vi "Charging_IPG Charging Status.vi"(8 "error in":errorcluster, 11 "MICS Dongle Address":refnum<visa-resource-name>="COM5") -> (0 "error out":errorcluster, 1 "IPG_ReceivedLevel":dbl=nan, 2 "TemperatureLevel":dbl=nan, 3 "ChargingState":string)   [LabVIEW 2010]
uses:
  Telemetry/Typedef Command List.ctl
panel:
  out "Charging Status":string
  out "ChargeWarning":dbl=nan
  # "Get Telemetry from IPG"
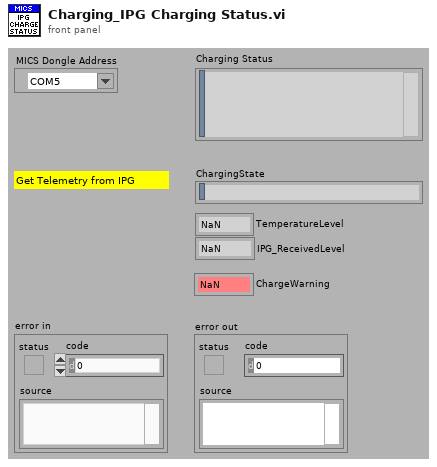
[diagram p1: front panel]
types:
  T1 = typedef "Typedef Command List.ctl" = enum16{"Get xPG Status", "xPG Stimulation", "Select Program", "Increment Program Amplitude", "Decrement Program Amplitude", "Get PoP Constants", "Get PPC Constants", "Get Program Names", "Set Pulse Amplitude", "Increment Pulse Amplitude", "Decrement Pulse Amplitude", "Get Pulse Widths", "Set Pulse Widths", "Increment Pulse Width", "Decrement Pulse Width", "Get Program Frequency", "Set Program Frequency", "Increment Program Frequency", "Decrement Program Frequency", "Inject Event", "Charging Control", "Get xPG Identity", "Set xPG Identity", "Restore Program Defaults", "Get Program Definition", "Set Program Definition", "Get Program Constants", "Set Program Constants", "Get Configurable Device Parameters", "Set Configurable Device Parameters", "Get Pulse Constants", "Set Pulse Constants", "Get Lead Limits", "Set Lead Limits", "Get Channel Calibrations", "Set Channel Calibrations", "<reserved 2>", "<reserved 3>", "<reserved 4>", "<reserved 5>", "<reserved 6>", "<reserved 7>", "Get Stim Asic HV Calibrations", "Set Stim Asic HV Calibrations", "<reserved 8>", "<reserved 9>", "Get CP Data", "Set CP Data", "Clear Log", "Read Log", "Append Log", "Get Patient Program Runtime", "Set Patient Program Runtime", "Impedance Measurement", "Enter Storage Mode", "Echo Short", "Echo Long", "Get General Calibration", "Set General Calibration", "Get Trim List", "Set Trim List", "Get Counter", "Set Counter", "Get Test Stimulation", "Set Test Stimulation", "Get Titration Stimulation", "Set Titration Stimulation", "Get Ramp Time", "Set Ramp Time", "Get VBAT", "Set Software Description Block", "Get Software Description Block", "Write Memory", "Read Memory", "Reset xPG", "Erase Flash Block", "Write Vectors", "Read Vectors", "Diagnostic Data", "Set Background Impedance", "Get Background Impedence ", "Set Test Waveform", "Calibrate Channel", "Get Log Range", "Reserved 0x55", "Reserved 0x56", "MICS Options", "Pair PPC", "Pair POP", "Stop Bootloader", "Tune MICS", "MICS Diagnostics", "Undefined"}
  T2 = cluster{"Command":T1, "Function":enum16{"Open Session", "Close Session", "Downlink Only", "Uplink Only", "Transceive (DN -> UP)"}, "MICS_ID":u32, "EXID":u32, "Use Local":bool, "Transceive Delay mS":dbl, "CP_DATA IN":u8[], "Parameters":string}
  T3 = enum16{"Open Session", "Close Session", "Downlink Only", "Uplink Only", "Transceive (DN -> UP)"}
  T4 = cluster{"Response Token":string, "Response Code":string, "bChecksum Valid":bool, "tChecksum Valid":bool, "CP_DATA OUT":u8[], "Data":string}
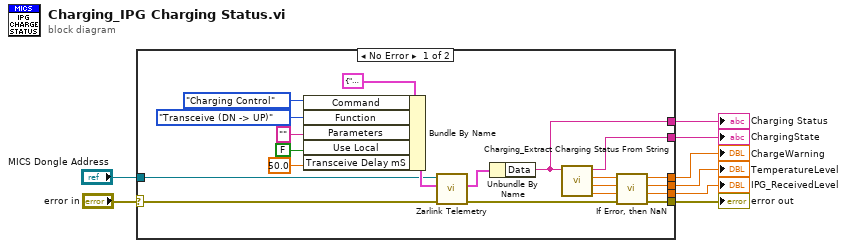
[diagram p0: block diagram]
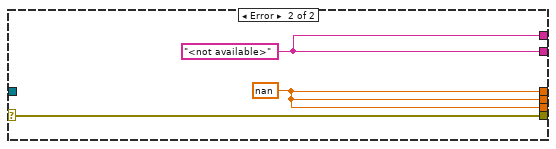
[diagram p2: hidden frame]
diagram:
  n1 = case shown="No Error" "error in" {
    selector: "error in" -> [w22 w31]
    tunnel: [w16 w31] -> w8
    tunnel: [w20 w29] -> w7
    tunnel: "MICS Dongle Address" -> [w19 _]
    tunnel: [w18 w29] -> w4
    tunnel: [w12 w30] -> w3
    tunnel: [w11 w30] -> w2
    tunnel: [w10 w30] -> w1
    frame No Error {
      n2 = Bundle By Name(cluster=T2 {"Command"=enum."Get xPG Status", "Function"=enum."Close Session", "MICS_ID"=0, "EXID"=16773121, "Use Local"=FALSE, "Transceive Delay mS"=100.0, "CP_DATA IN"=[], "Parameters"=""} ("Input"), "Command"=Typedef_Command_List."Charging Control", "Function"=T3."Transceive (DN -> UP)", "Parameters"="", "Use Local"=FALSE, "Transceive Delay mS"=50.0) -> (w28:T2)
      n3 = call "Zarlink Telemetry.vi"("error in (no error)"=w22, "Input"=w28, "MICS Dongle Address"=w19) -> ("error out"=w17:errorcluster, "Output"=w24:T4)  [unwired: 6 in, 1 out]
      n4 = Unbundle By Name(w24) -> ("Data"=w18:string)
      n5 = call "Charging_Extract Charging Status From String.vi"("Charging Status"=w18) -> ("IPG_ReceivedLevel"=w15:dbl, "TemperatureLevel"=w14:dbl, "ChargeWarning"=w13:dbl, "ChargingState"=w20:string)  [unwired: 7 in]
      n6 = call "If Error, then NaN.vi"("error in (T)"=w17, "value3"=w15, "value2"=w14, "value1"=w13) -> ("error out"=w16:errorcluster, "value out3"=w12:dbl, "value out2"=w11:dbl, "value out1"=w10:dbl)  [unwired: 2 in]
    }
    frame Error {
      w29 = "<not available>" ("ChargingState")
      w30 = nan ("ChargeWarning")
    }
  }
  "error out" <- w8
  "ChargingState" <- w7
  "ChargeWarning" <- w1
  "TemperatureLevel" <- w2
  "IPG_ReceivedLevel" <- w3
  "Charging Status" <- w4
